vi "Get Attribute Name and Parent ID.vi"(8 "error in (no error)":errorcluster, 10 "Tag":string, 11 "ITest Executive in":refnum<class "ITest Executive.lvclass">) -> (0 "error out":errorcluster, 1 "Attribute Name":string, 2 "Parent ID":string, 3 "ITest Executive out":refnum<class "ITest Executive.lvclass">)   [LabVIEW 2020, in "Test Executive.lvlib" / "ITest Executive.lvclass"]
uses:
  <vilib>/gpm_packages/@cs/test-executive/Source/Test Executive/ITestExecutive/ITest Executive.lvclass
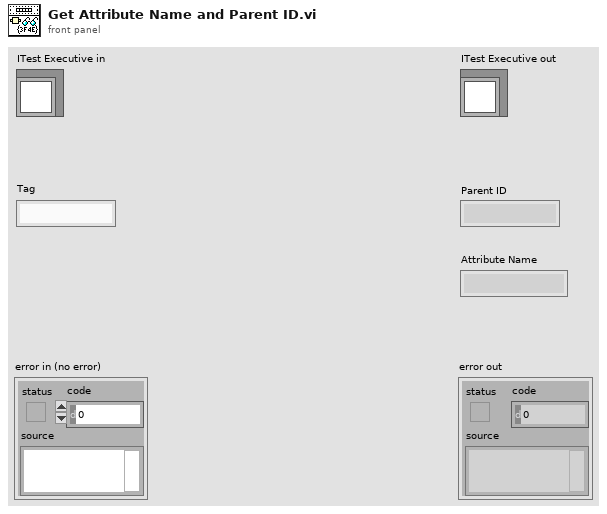
[diagram p1: front panel]
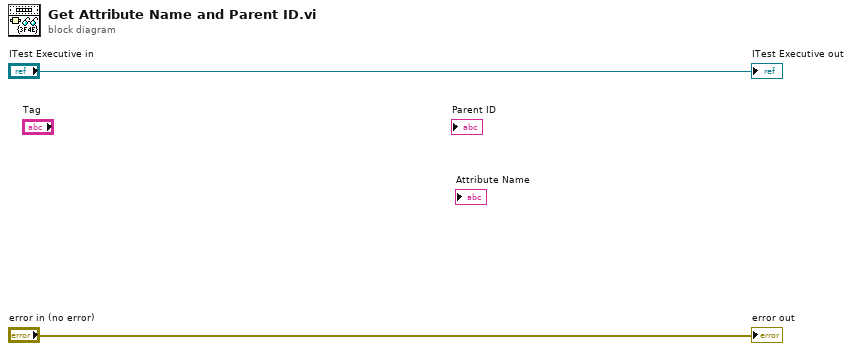
[diagram p0: block diagram]
diagram:
  "error out" <- "error in (no error)"
  "ITest Executive out" <- "ITest Executive in"
